vi "LanchSpeedAndAngleCalculator.vi"(2 "g":dbl=9.82, 3 "b":dbl=60.0, 4 "h":dbl, 5 "d":dbl) -> (0 "V":dbl, 1 "a":dbl)   [LabVIEW 2011]
uses:
  <vilib>/express/express arith-compare/Formula/XNode/ExpressFormulaBlockNode.xnode
panel:
  out "Numeric":ext[unit]=6.6741999999999999998e-11 format="%#.4g"
  # "a - degrees\nb - degrees\nh - meters\nd - meters\ng - m/s^2\nV - m/s"
  # "b"
  # "V"
  # "h"
  # "a"
  # "d"
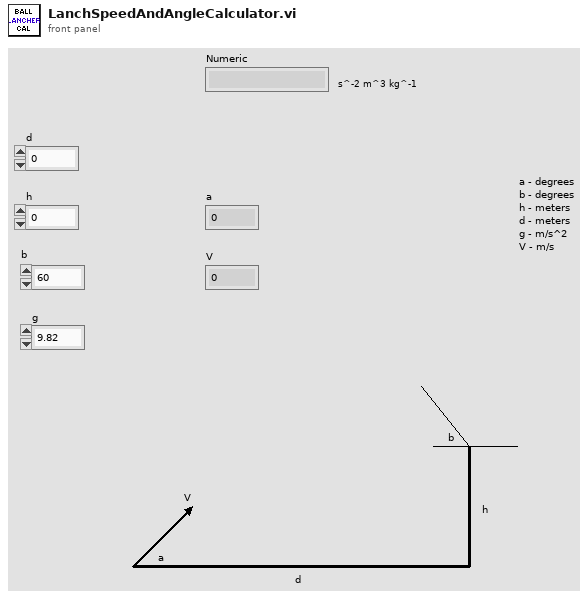
[diagram p1: front panel]
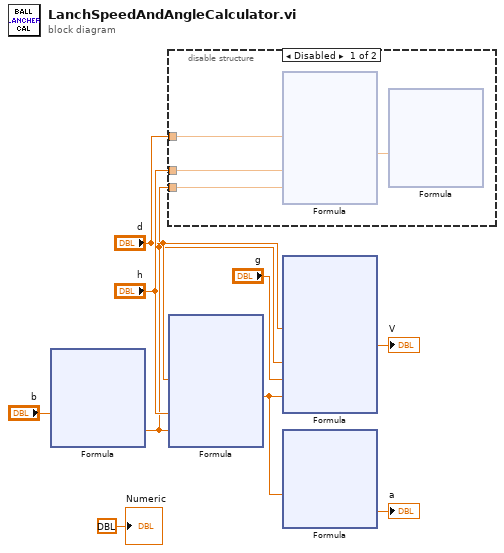
[diagram p0: block diagram]
diagram:
  n1 = xnode "Formula"("b"="b") -> ("Result"=w2:dbl)  [unwired: 1 in, 1 out]
  n2 = disable-structure shown="Disabled" {
    disable-tunnel: "d" -> [w13 _]
    disable-tunnel: "h" -> [w12 _]
    disable-tunnel: w2 -> [w11 _]
    frame Disabled {
      n3 = xnode "Formula"("d"=w13, "h"=w12, "b"=w11) -> ("Result"=w10:dbl)  [unwired: 1 in, 1 out]
      n4 = xnode "Formula"("r"=w10) -> ()  [unwired: 1 in, 2 out]
    }
    frame Enabled {
    }
  }
  n5 = xnode "Formula"("d"="d", "h"="h", "b"=w2) -> ("Result"=w4:dbl)  [unwired: 1 in, 1 out]
  n6 = xnode "Formula"("d"="d", "b"=w2, "g"="g", "a"=w4) -> ("Result"=→"V":dbl)  [unwired: 1 in, 1 out]
  n7 = xnode "Formula"("r"=w4) -> ("Result"=→"a":dbl)  [unwired: 1 in, 1 out]
  "Numeric" <- ext[unit] 6.6741999999999999998e-11
